vi "LVClass_HasoSlopes Apply NeighborExtension.vi"(0 "HasoSlopes in":refnum<class "HasoSlopes.lvclass">, 11 "error in (no error)":errorcluster) -> (4 "HasoSlopes out":refnum<class "HasoSlopes.lvclass">, 15 "error out":errorcluster)   [LabVIEW 2020, in "HasoSlopes.lvclass"]
uses:
  HasoSlopes.lvclass
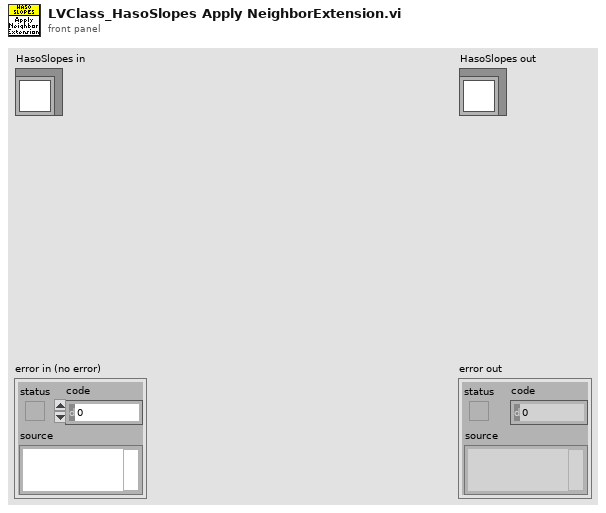
[diagram p1: front panel]
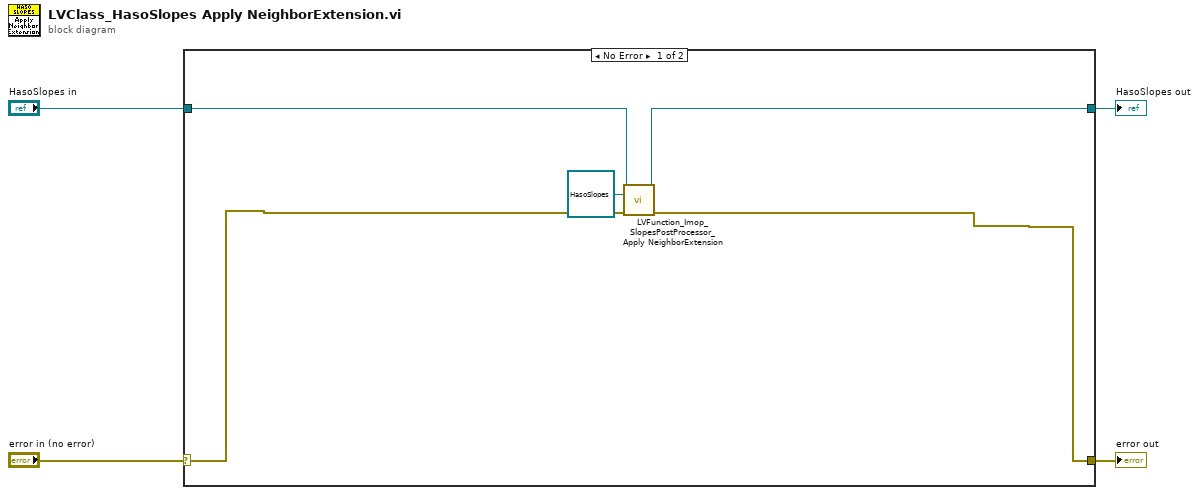
[diagram p0: block diagram]
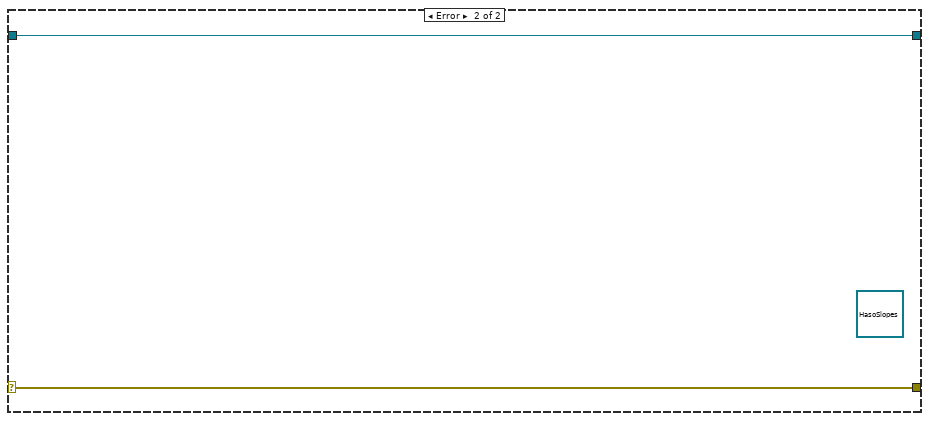
[diagram p2: hidden frame]
diagram:
  n1 = case shown="No Error" "error in (no error)" {
    selector: "error in (no error)" -> [w9 w11]
    tunnel: [w8 w11] -> w3
    tunnel: [w6 w10] -> w1
    tunnel: "HasoSlopes in" -> [w7 w10]
    frame No Error {
      n2 = call "LVFunction_Imop_SlopesPostProcessor_Apply NeighborExtension.vi"("HasoSlopes in"=w7, "HasoSlopes OUT"=refnum<class "HasoSlopes.lvclass"> refnum, "error in (no error)"=w9) -> ("HasoSlopes out"=w6:refnum<class "HasoSlopes.lvclass">, "error out"=w8:errorcluster)  [unwired: 10 in, 1 out]
    }
    frame Error {
      (unwired) refnum<class "HasoSlopes.lvclass"> refnum ("HasoSlopes OUT")
    }
  }
  "error out" <- w3
  "HasoSlopes out" <- w1
